vi "Start Command.vi"(8 "error in (no error)":errorcluster, 9 "Command Name":string, 10 "Robot Actors.lvlib:Command.lvlib:Command.lvclass":refnum<class "Command.lvclass">, 11 "Running Command in":refnum<class "Running Command.lvclass">) -> (0 "error out":errorcluster, 3 "Running Command out":refnum<class "Running Command.lvclass">)   [LabVIEW 2014, in "Robot Actors.lvlib" / "Command Processor.lvlib" / "Running Command.lvclass"]
uses:
  Running Command.lvclass
  Command/Command Class/Command.lvclass
  <vilib>/ActorFramework/Message Enqueuer/Message Enqueuer.lvclass/Message Enqueuer.ctl
  <vilib>/ActorFramework/Message Enqueuer/Enqueue.vi
  <vilib>/ActorFramework/Message Priority Queue/Priority Enqueue.vi
  <vilib>/ActorFramework/Stop Msg/Stop Msg.lvclass
  Command Processor Class/Command Processor.lvclass
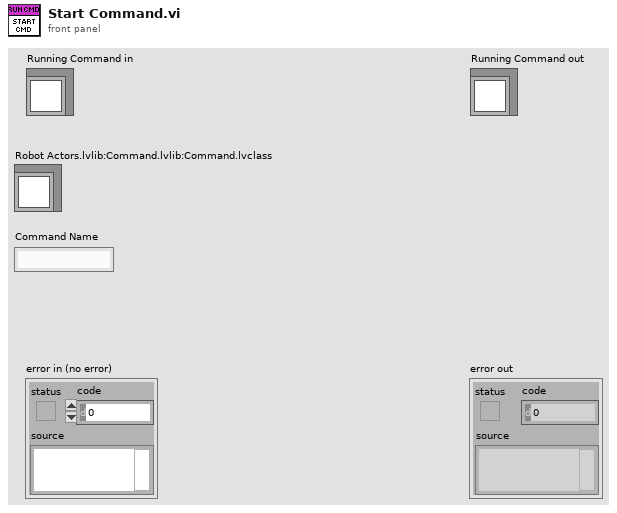
[diagram p1: front panel]
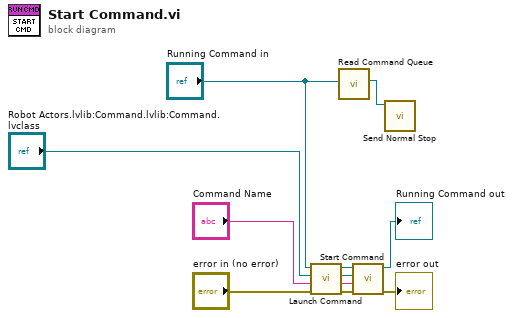
[diagram p0: block diagram]
diagram:
  n1 = call-dynamic "Launch Command.vi"("error in (no error)"="error in (no error)", "Command Name In"="Command Name", "Command In"="Robot Actors.lvlib:Command.lvlib:Command.lvclass", "Command Processor in"="Running Command in") -> ("error out"=w5:errorcluster, "Command Name Out"=w6:string, "Command Out"=w7:refnum<class "Command.lvclass">, "Command Processor out"=w8:refnum<class "Running Command.lvclass">)  [unwired: 4 in]
  n2 = call-dynamic "Read Command Queue.vi"("Command Processor in"="Running Command in") -> ("Actor Framework:Message Enqueuer"=w1:refnum<class "Message Enqueuer.lvclass">)  [unwired: 8 in, 2 out]
  n3 = call-parent "Start Command.vi"("error in (no error)"=w5, "Command Name"=w6, "Robot Actors.lvlib:Command.lvlib:Command.lvclass"=w7, "Command Processor in"=w8) -> ("error out"=→"error out":errorcluster, "Command Processor out"=→"Running Command out":refnum<class "Running Command.lvclass">)  [unwired: 6 in]
  n4 = call <vilib>:"Send Normal Stop.vi"("Message Enqueuer"=w1) -> ()  [unwired: 10 in, 1 out]
